vi "Step Update Test Parameters.vi"(8 "error in (no error)":errorcluster, 10 "Test Parameters":variant, 11 "Test_ID (\"\")":string) -> (0 "error out":errorcluster, 3 "Parameter String":string)   [LabVIEW 2011]
uses:
  www/tests/Test Function.ctl
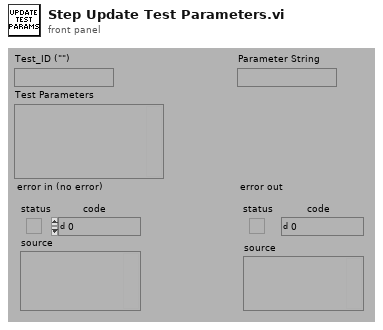
[diagram p1: front panel]
types:
  T1 = typedef "Test Function.ctl" = enum16{"Test Config", "Test Storage", "Test Pre-Process", "Unflatten Test Parameters", "Flatten Test Parameters"}
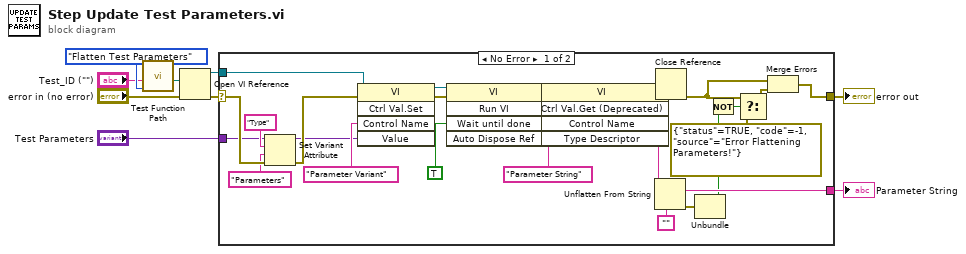
[diagram p0: block diagram]
diagram:
  n1 = call "Test Function Path.vi"("Object Type (Test Config)"=Test_Function."Flatten Test Parameters", "Object Name (\"\")"="Test_ID (\"\")") -> ("Object Path"=w7:path)  [unwired: 1 in, 8 out]
  n2 = Open VI Reference(vi path=w7, error in (no error)="error in (no error)") -> (vi reference=w5:refnum<vi>, error out=w4:errorcluster)  [unwired: 1 in, 3 out]
  n3 = case shown="No Error" w4 {
    selector: w4 -> [w18 w36]
    tunnel: w5 -> [w35 _]
    tunnel: [w26 w36] -> w9
    tunnel: [w27 _] -> w8
    tunnel: "Test Parameters" -> [w13 _]
    frame No Error {
      n4 = Set Variant Attribute(Variant=w13, name="Type", value="Parameters" ("name"), error in=w18) -> (Variant out=w15:variant, error out=w17:errorcluster)  [unwired: 1 out]
      n5 = invoke class="VI" method="Ctrl Val.Set"(reference=w35, error in=w17, "Control Name"="Parameter Variant", "Value"=w15) -> (reference out=w10:refnum<vi>, error out=w11:errorcluster)  [unwired: 1 in, 3 out]
      n6 = invoke class="VI" method="Run VI"(reference=w10, error in=w11, "Wait until done"=TRUE) -> (reference out=w31:refnum<vi>, error out=w32:errorcluster)  [unwired: 2 in, 3 out]
      n7 = invoke class="VI" method="Ctrl Val.Get (Deprecated)"(reference=w31, error in=w32, "Control Name"="Parameter String") -> (reference out=w28:refnum<vi>, error out=w29:errorcluster, "Get Control Value"=w30:string)  [unwired: 2 in, 2 out]
      n8 = Unflatten From String(type="", binary string=w30) -> (value=w27:string, error out=w20:errorcluster)  [unwired: 1 in, 3 out]
      n9 = Close Reference(reference=w28, error in (no error)=w29) -> (error out=w23:errorcluster)
      n10 = Unbundle(w20) -> ("status"=w22:bool)  [unwired: 2 out]
      n11 = Not(x=w22) -> (.not. x?=w21:bool)
      n12 = Select(t=w23, s=w21, f=errorcluster {"status"=TRUE, "code"=-1, "source"="Error Flattening Parameters!"}) -> (s? t:f=w24:errorcluster)
      n13 = Merge Errors(w23, w24) -> (w26:errorcluster)
    }
    frame Error {
    }
  }
  "error out" <- w9
  "Parameter String" <- w8
